vi "Last Points.vi"(1 "Ring Buffers":T1) -> (0 "Latest Points":dbl[](array[numeric]))   [LabVIEW 2012, in "Collection.lvclass"]
doc: "Returns the most recent values from the ring buffers in a collection."
uses:
  Collection.lvclass
  Readable/TX Graph.ctl
  Readable/Readable.lvclass
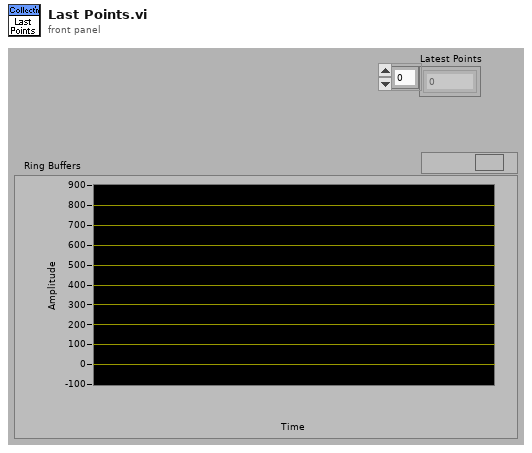
[diagram p1: front panel]
types:
  T1 = typedef "Readable.lvclass/TX Graph.ctl" = cluster{"Data Points":cluster{"t":timestamp, "x":dbl}[]}[]
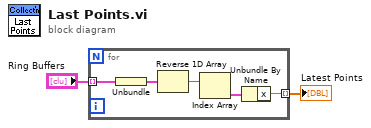
[diagram p0: block diagram]
diagram:
  n1 = for {
    tunnel: "Ring Buffers" -> [w7] mode=indexing
    tunnel: [w3] -> w1 mode=indexing
    n2 = Unbundle(w7) -> ("Data Points"=w6:cluster{"t":timestamp, "x":dbl}[])
    n3 = Reverse 1D Array(array=w6) -> (reversed array=w5:cluster{"t":timestamp, "x":dbl}[])
    n4 = Index Array(array=w5) -> (element=w4:cluster{"t":timestamp, "x":dbl})  [unwired: 1 in]
    n5 = Unbundle By Name(w4) -> ("x"=w3:dbl)
  }
  "Latest Points" <- w1
